vi "Calor Combustión.vi"() -> ()   [LabVIEW 2021]
panel:
  in  "Sustancia":u16(ring) items=["Etanol", "Metano, default", "Butano", "Propano"]
  in  "stop":bool
  out "Entalpia Reaccion CombustionIncompleta":dbl
  out "Entalpia R. Combustion Completa":dbl
  out "Entalpia \nReacción":dbl
  in  "Porcentaje de Combustión":dbl(slide) scale=0.0..100.0
  in  "Masa":dbl
  # "CALOR DE COMBUSTION"
  # "gr"
  # "kJ"
  # "Desarrollado por:\n     Cesar Augusto Quiñones Segura\n     Andrea Carolina Sanchez Diaz\n     Jhon Erik Navarrete Gómez"
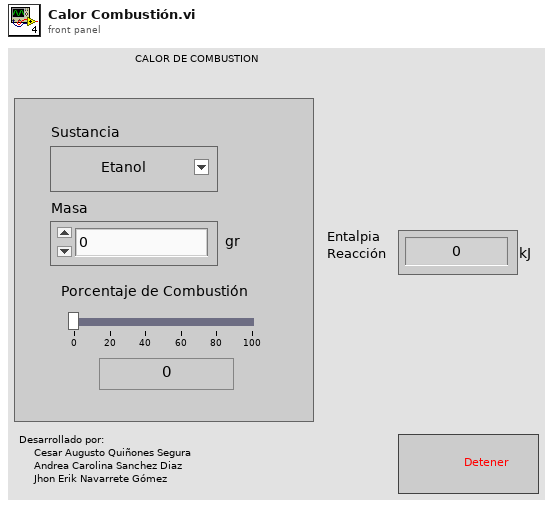
[diagram p1: front panel]
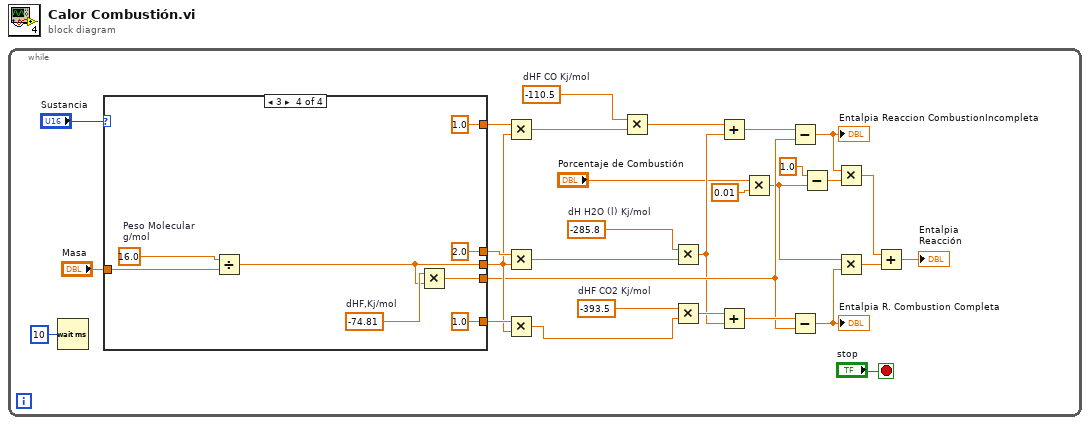
[diagram p0: block diagram]
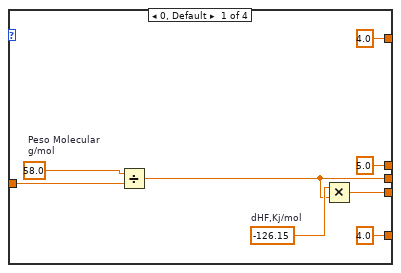
[diagram p2: hidden frame]
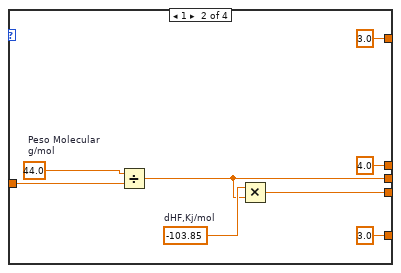
[diagram p3: hidden frame]
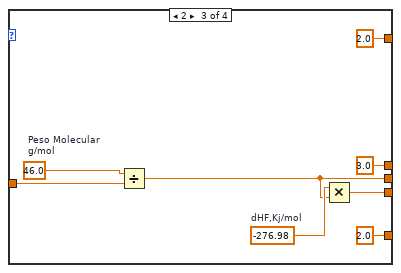
[diagram p4: hidden frame]
diagram:
  n1 = while {
    stop <- "stop" stop-if-true
    w22 = -285.8  # dH H2O (l) Kj/mol
    w24 = -110.5  # dHF CO Kj/mol
    w26 = -393.5  # dHF CO2 Kj/mol
    n2 = Wait (ms)(milliseconds to wait=u32 10) -> ()  [unwired: 1 out]
    n3 = case shown="3" "Sustancia" {
      tunnel: "Masa" -> [w36 w45 w52 w60]
      tunnel: [4.0 3.0 2.0 1.0] -> w29
      tunnel: [4.0 3.0 2.0 1.0] -> w28
      tunnel: [5.0 4.0 3.0 2.0] -> w27
      tunnel: [w35 w40 w51 w58] -> w15
      tunnel: [w31 w39 w48 w59] -> w16
      frame 0, Default {
        w38 = 58.0  # Peso Molecular  g/mol
        w37 = -126.15  # dHF,Kj/mol
        n4 = Divide(x=w38, y=w36) -> (x/y=w31:dbl)
        n5 = Multiply(x=w37, y=w31) -> (x*y=w35:dbl)
      }
      frame 1 {
        w46 = 44.0  # Peso Molecular  g/mol
        w41 = -103.85  # dHF,Kj/mol
        n6 = Divide(x=w46, y=w45) -> (x/y=w39:dbl)
        n7 = Multiply(x=w41, y=w39) -> (x*y=w40:dbl)
      }
      frame 2 {
        w54 = 46.0  # Peso Molecular  g/mol
        w53 = -276.98  # dHF,Kj/mol
        n8 = Divide(x=w54, y=w52) -> (x/y=w48:dbl)
        n9 = Multiply(x=w53, y=w48) -> (x*y=w51:dbl)
      }
      frame 3 {
        w62 = 16.0  # Peso Molecular  g/mol
        w61 = -74.81  # dHF,Kj/mol
        n10 = Divide(x=w62, y=w60) -> (x/y=w59:dbl)
        n11 = Multiply(x=w61, y=w59) -> (x*y=w58:dbl)
      }
    }
    n12 = Multiply(x=w28, y=w16) -> (x*y=w23:dbl)
    n13 = Multiply(x=w27, y=w16) -> (x*y=w21:dbl)
    n14 = Multiply(x=w29, y=w16) -> (x*y=w25:dbl)
    n15 = Multiply(x=w24, y=w23) -> (x*y=w17:dbl)
    n16 = Multiply(x=w22, y=w21) -> (x*y=w7:dbl)
    n17 = Multiply(x=w26, y=w25) -> (x*y=w20:dbl)
    n18 = Add(x=w17, y=w7) -> (x+y=w18:dbl)
    n19 = Add(x=w20, y=w7) -> (x+y=w19:dbl)
    n20 = Multiply(x="Porcentaje de Combustión", y=0.01) -> (x*y=w3:dbl)
    n21 = Subtract(x=w18, y=w15) -> (x-y=w12:dbl)
    "Entalpia Reaccion CombustionIncompleta" <- w12
    n22 = Subtract(x=w19, y=w15) -> (x-y=w13:dbl)
    "Entalpia R. Combustion Completa" <- w13
    n23 = Subtract(x=1.0, y=w3) -> (x-y=w11:dbl)
    n24 = Multiply(x=w12, y=w11) -> (x*y=w9:dbl)
    n25 = Multiply(x=w3, y=w13) -> (x*y=w8:dbl)
    n26 = Add(x=w9, y=w8) -> (x+y=→"Entalpia \nReacción":dbl)
  }
